vi "Get Loop Assignment.vi"(8 "error in (no error)":errorcluster, 11 "Module in":refnum<class "Module.lvclass">) -> (0 "error out":errorcluster, 2 "Loop Assignment":string, 3 "Module out":refnum<class "Module.lvclass">)   [LabVIEW 2019, in "Module.lvclass"]
uses:
  Module.lvclass
  Module Configuration.ctl
  Module.lvclass/Module.ctl
  VI/Module Loop/Module Loop.lvclass
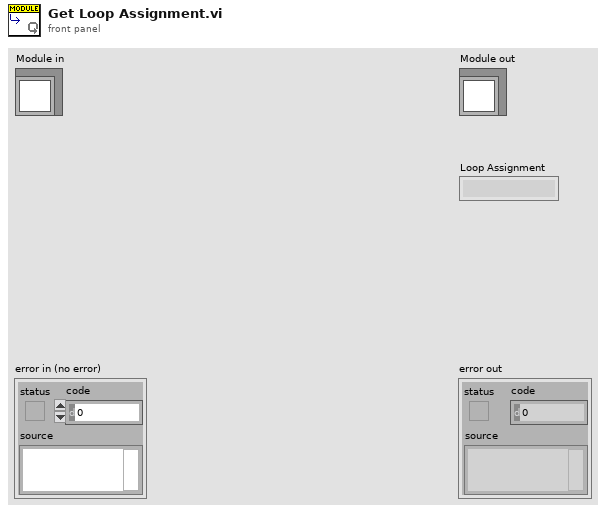
[diagram p1: front panel]
types:
  T1 = typedef "Module Loop.lvclass/Module Configuration.ctl" = cluster{"Type":string, "Direction":string, "Speed":string, "Channels":string, "FXP Type":string}
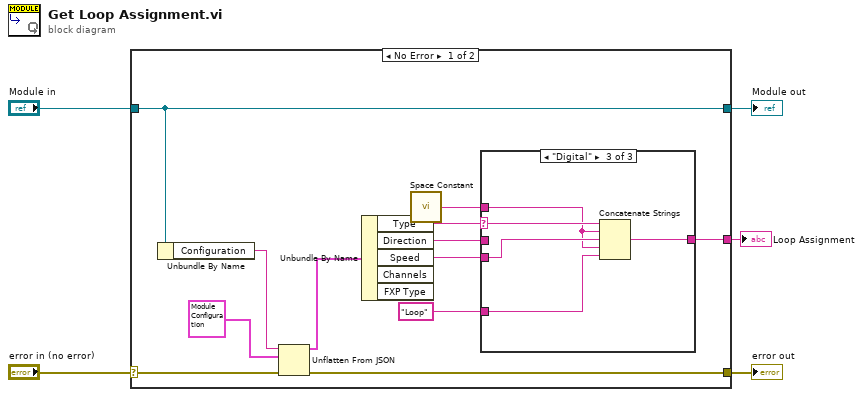
[diagram p0: block diagram]
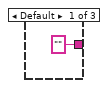
[diagram p2: hidden frame]
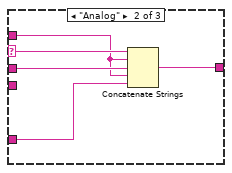
[diagram p3: hidden frame]
diagram:
  n1 = case shown="No Error" "error in (no error)" {
    selector: "error in (no error)" -> [w13 w30]
    tunnel: [w12 w30] -> w4
    tunnel: [w14 w29] -> w2
    tunnel: "Module in" -> [w14 w29]
    tunnel: [w7 _] -> w1
    frame No Error {
      n2 = Unbundle By Name(w14) -> ("Configuration"=w17:string)
      n3 = Unflatten From JSON(JSON string=w17, type and defaults=T1 {"Type"="Digital", "Direction"="Input", "Speed"="High Speed", "Channels"="8", "FXP Type"=""} ("Cluster"), error in (no error)=w13) -> (value=w15:T1, error out=w12:errorcluster)  [unwired: 4 in]
      n4 = Unbundle By Name(w15) -> ("Type"=w11:string, "Direction"=w10:string, "Speed"=w8:string)  [unwired: 2 out]
      n5 = call <vilib>:"Space Constant.vi"() -> ("String"=w6:string)
      n6 = case shown="\"Digital\"" w11 {
        selector: w11 -> [_ w23 w28]
        tunnel: w10 -> [_ w22 _]
        tunnel: "Loop" ("string") -> [_ w21 w27]
        tunnel: ["" w20 w26] -> w7
        tunnel: w8 -> [_ _ w25]
        tunnel: w6 -> [_ w19 w24]
        frame Default {
        }
        frame "Analog" {
          n7 = Concatenate Strings(w23, w19, w22, w19, w21) -> (w20:string)
        }
        frame "Digital" {
          n8 = Concatenate Strings(w28, w24, w25, w24, w27) -> (w26:string)
        }
      }
    }
    frame Error {
    }
  }
  "error out" <- w4
  "Module out" <- w2
  "Loop Assignment" <- w1
